vi "Camer Control Variables.vi"() -> ()   [LabVIEW 2014]
panel:
  out "Number of Images in Set":i32
  out "Camera Trigger Command":bool
  in  "Half Capture Time":u32=750
  in  "Force Capturing":bool
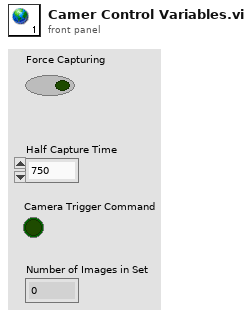
[diagram p1: front panel]
diagram:
